vi "Can Destroy.vi"(8 "Error in":errorcluster, 10 "Actor in":refnum<class "Actor.lvclass">) -> (1 "Destroy":bool, 2 "Actor out":refnum<class "Actor.lvclass">)   [LabVIEW 2025, in "jettl.lvlib" / "Actor.lvlib"]
uses:
  Actor.lvlib
  Actor/Actor.lvclass
  Destroy Msg/Destroy Msg.lvlib
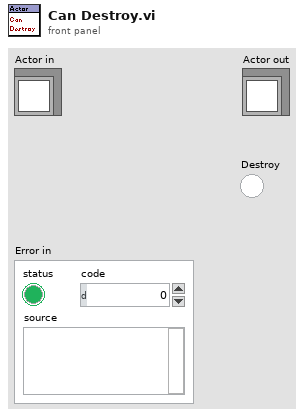
[diagram p1: front panel]
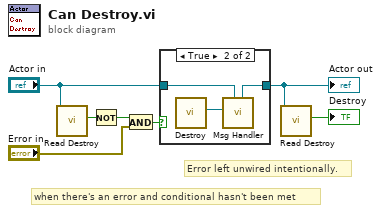
[diagram p0: block diagram]
diagram:
  # "Error left unwired intentionally."
  # "when there's an error and conditional hasn't been met"
  n1 = call-dynamic "Read Destroy.vi"("Actor in"="Actor in") -> ("Destroy"=w3:bool)  [unwired: 10 in]
  n2 = Not(x=w3) -> (.not. x?=w7:bool)
  n3 = And(x=w7, y="Error in") -> (x .and. y?=w6:bool)
  n4 = case shown="True" w6 {
    tunnel: [w8 w10] -> w2
    tunnel: "Actor in" -> [w8 w11]
    frame False {
    }
    frame True {
      n5 = call "Destroy.vi"() -> ("Msg"=w9:refnum<class "Msg.lvclass">)  [unwired: 11 in]
      n6 = call "Msg Handler.vi"("Actor in"=w11, "Msg"=w9) -> ("Actor out"=w10:refnum<class "Actor.lvclass">)  [unwired: 8 in, 1 out]
    }
  }
  "Actor out" <- w2
  n7 = call-dynamic "Read Destroy.vi"("Actor in"=w2) -> ("Destroy"=→"Destroy":bool)  [unwired: 10 in]
